vi "RT Module ID.vi"(0 "Module ID In":i32, 2 "HW Name":T1, 11 "error in":errorcluster, 13 "Action":T2) -> (4 "Module Id Out":i32, 8 "All HW Name Out":T1[](array[typedef]), 10 "All HW-ID Out":i32[](array[numeric]), 15 "error out":errorcluster)   [LabVIEW 2024]
uses:
  Host-Control's/HW Name Enum.ctl
  Host-Control's/Module ID Action Enum.ctl
  13ccd86a-bc50-4ded-b990-c72d3f23a435.vi
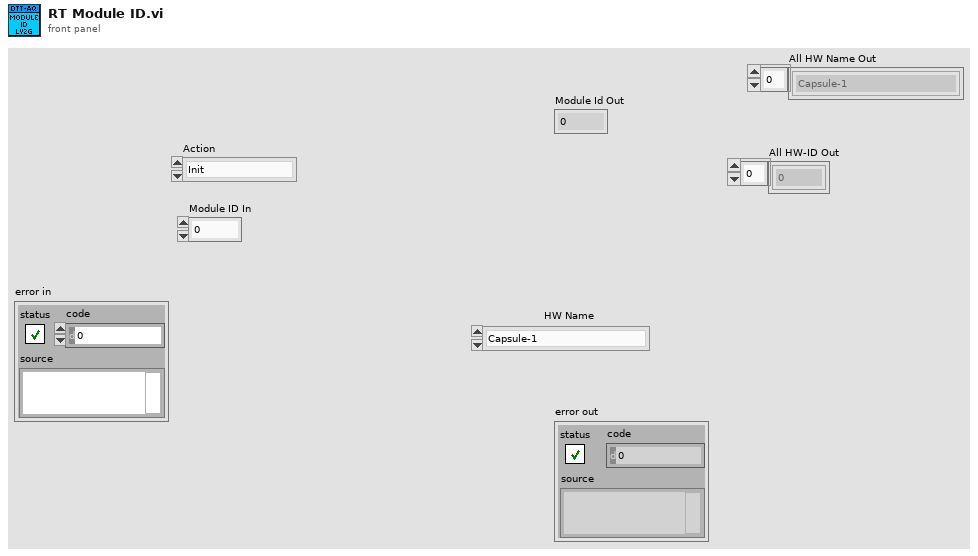
[diagram p1: front panel]
types:
  T1 = typedef "HW Name Enum.ctl" = enum16{"Capsule-1", "Capsule-2", "Capsule-3", "Capsule-4", "sb-RIO", "Safety", "Release"}
  T2 = typedef "Module ID Action Enum.ctl" = enum16{"Init", "Insert", "Get a ID", "Get all ID"}
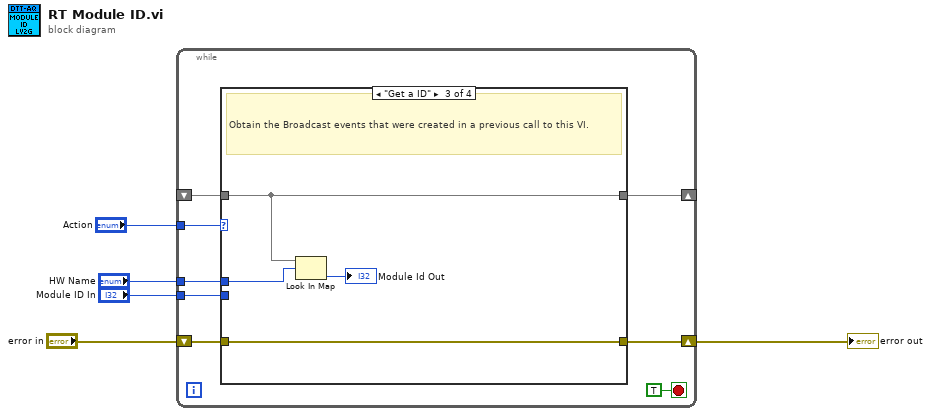
[diagram p0: block diagram]
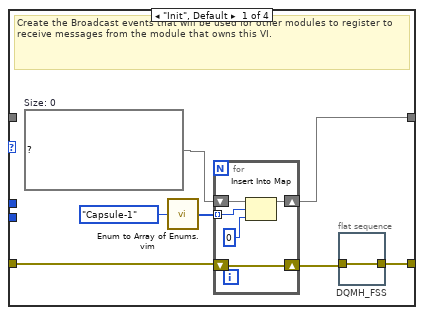
[diagram p2: hidden frame]
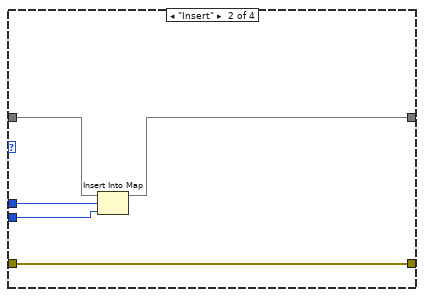
[diagram p3: hidden frame]
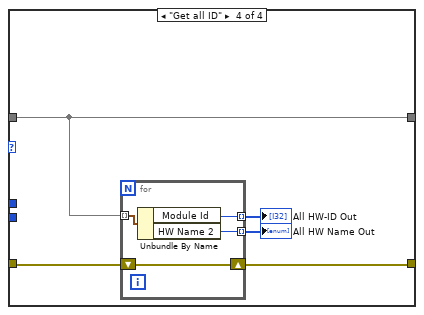
[diagram p4: hidden frame]
diagram:
  n1 = while {
    tunnel: "HW Name" -> [w11]
    tunnel: "Module ID In" -> [w10]
    tunnel: "Action" -> [w9]
    shift-right: [w13] -> w5
    shift-left: "error in" -> [w12]
    shift-right: [w7] -> _
    shift-left: _ -> [w6]
    stop <- TRUE stop-if-true
    n2 = case shown="\"Get a ID\"" w9 {
      tunnel: [w19 w27 w33 w40] -> w13
      tunnel: w12 -> [w17 w27 w33 w39]
      tunnel: [w20 w30 w35 w37] -> w7
      tunnel: w6 -> [_ w31 w35 w37]
      tunnel: w11 -> [_ w29 w32 _]
      tunnel: w10 -> [_ w28 _ _]
      frame "Init", Default {
        w15 = map{T1, i32} {}  # Size: 0
        # "Create the Broadcast events that will be used for other modules to register to receive messages from the module that owns this VI."
        n3 = call "Enum to Array of Enums.vim"("enum"=HW_Name_Enum."Capsule-1" ("HW Name")) -> ("array of enums"=w16:T1[])
        n4 = for {
          shift-right: [w25] -> w20
          shift-left: w15 -> [w24]
          shift-right: [w23] -> w18
          shift-left: w17 -> [w23]
          tunnel: w16 -> [w22] mode=indexing
          n5 = Insert Into Map(map in=w24, key=w22, value=0) -> (map out=w25:map{T1, i32})  [unwired: 2 out]
        }
        n6 = flat-sequence "DQMH_FSS" {
          tunnel: [w26] -> w19
          tunnel: w18 -> [w26]
          frame #0 {
          }
        }
      }
      frame "Insert" {
        n7 = Insert Into Map(map in=w31, key=w29, value=w28) -> (map out=w30:map{T1, i32})  [unwired: 2 out]
      }
      frame "Get a ID" {
        # "Obtain the Broadcast events that were created in a previous call to this VI."
        n8 = Look In Map(map=w35, key=w32) -> (value=→"Module Id Out":i32)  [unwired: 1 in, 1 out]
      }
      frame "Get all ID" {
        n9 = for {
          tunnel: w37 -> [w44] mode=indexing
          tunnel: [w43] -> w38 mode=indexing
          shift-right: [w42] -> w40
          shift-left: w39 -> [w42]
          tunnel: [w41] -> w36 mode=indexing
          n10 = Unbundle By Name(w44) -> ("Module Id"=w43:i32, "HW Name 2"=w41:T1)
        }
        "All HW-ID Out" <- w38
        "All HW Name Out" <- w36
      }
    }
  }
  "error out" <- w5
